vi "SubVI Tester.vi"() -> ()   [LabVIEW 2015]
uses:
  Weather Data.ctl
panel:
  out "Weather Data Out":T1={"Current Temperature"=0.0, "Max Temperature"=0.0, "Min Temperature"=0.0, "Warning?"=FALSE, "Warning Text"="No Warning", "Units"=enum."Fahrenheit"}
  in  "Min Temperature":dbl=10.0
  in  "Max Temperature":dbl=30.0
  in  "Stop":bool
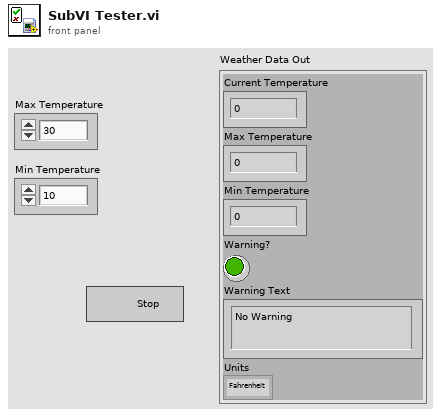
[diagram p1: front panel]
types:
  T1 = typedef "Weather Data.ctl" = cluster{"Current Temperature":dbl, "Max Temperature":dbl, "Min Temperature":dbl, "Warning?":bool, "Warning Text":string, "Units":enum16{"Fahrenheit", "Celsius"}}
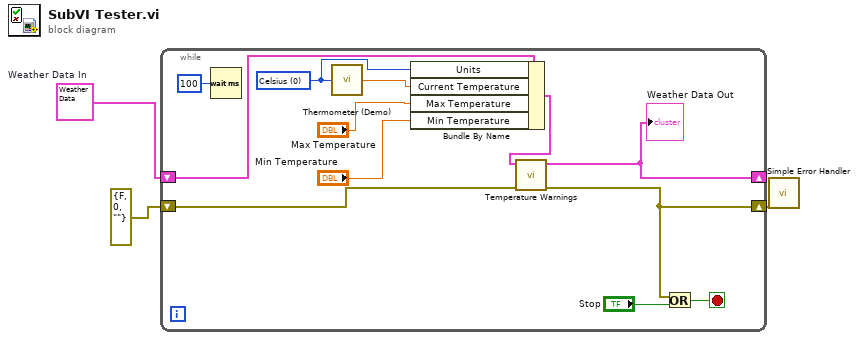
[diagram p0: block diagram]
diagram:
  w1 = T1 {"Current Temperature"=29.937499999999993, "Max Temperature"=30.0, "Min Temperature"=10.0, "Warning?"=FALSE, "Warning Text"="No Warning", "Units"=enum."Fahrenheit"}  # Weather Data In
  n1 = while {
    shift-right: [w11] -> w3
    shift-left: errorcluster {"status"=FALSE, "code"=0, "source"=""} ("error out") -> [w12]
    shift-right: [w7] -> _
    shift-left: w1 -> [w5]
    stop <- w13 stop-if-true
    w4 = u16 0 items=["Celsius", "Fahrenheit"] ("Units (0: Celsius)")
    n2 = Wait (ms)(milliseconds to wait=u32 100) -> ()  [unwired: 1 out]
    n3 = call "Thermometer (Demo).vi"("Units (0: Celsius)"=w4) -> ("Temperature Value"=w10:dbl)
    n4 = Bundle By Name(cluster=w5, "Units"=w4, "Current Temperature"=w10, "Max Temperature"="Max Temperature", "Min Temperature"="Min Temperature") -> (w6:T1)
    n5 = call "Temperature Warnings.vi"("Error In"=w12, "Weather Data In"=w6) -> ("Error Out"=w11:errorcluster, "Weather Data 2 Out"=w7:T1)  [unwired: 8 in]
    "Weather Data Out" <- w7
    n6 = Or(x=w11, y="Stop") -> (x .or. y?=w13:bool)
  }
  n7 = call <vilib>:"Simple Error Handler.vi"("error in (no error)"=w3) -> ()  [unwired: 4 in, 5 out]
